vi "set_value.vi"(8 "error in (no error)":errorcluster, 9 "value":variant, 10 "key":string, 11 "Map.lvclass in":refnum<class "Map.lvclass">) -> (0 "error out":errorcluster, 3 "Map.lvclass out":refnum<class "Map.lvclass">)   [LabVIEW 2010, in "Map.lvclass"]
doc: "This method assigns a value to a given key. You can access only direct entry, but not entries further down the hierarchy in the case of a nested map."
uses:
  Map.lvclass
  element_cluster.ctl
  Map.lvclass/Map.ctl
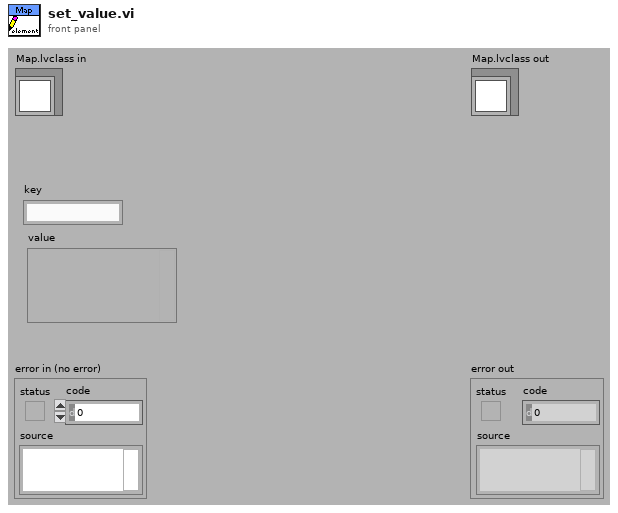
[diagram p1: front panel]
types:
  T1 = typedef "Map.lvclass/element_cluster.ctl" = cluster{"key":string, "value":variant}
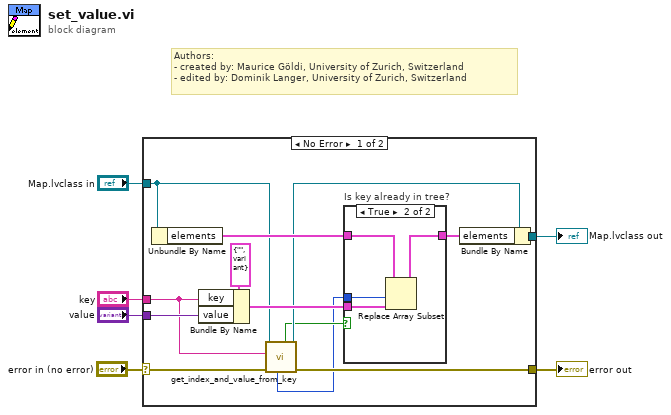
[diagram p0: block diagram]
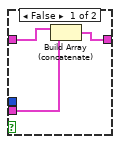
[diagram p2: hidden frame]
diagram:
  # "Authors: \n- created by: Maurice Göldi, University of Zurich, Switzerland\n- edited by: Dominik Langer, University of Zurich, Switzerland"
  n1 = case shown="No Error" "error in (no error)" {
    selector: "error in (no error)" -> [w13 w27]
    tunnel: [w12 w27] -> w5
    tunnel: [w19 w28] -> w3
    tunnel: "Map.lvclass in" -> [w10 w28]
    tunnel: "key" -> [w11 _]
    tunnel: "value" -> [w15 _]
    frame No Error {
      n2 = Unbundle By Name(w10) -> ("elements"=w18:T1[])
      n3 = Bundle By Name(cluster=T1 {"key"="", "value"=variant} ("map_elements"), "key"=w11, "value"=w15) -> (w14:T1)
      n4 = call "get_index_and_value_from_key.vi"("error in (no error)"=w13, "key"=w11, "Map.lvclass in"=w10) -> ("error out"=w12:errorcluster, "Map.lvclass out"=w9:refnum<class "Map.lvclass">, "key exists?"=w8:bool, "index"=w7:i32)  [unwired: 5 out]
      n5 = case "Is key already in tree?" shown="True" w8 {
        tunnel: w18 -> [w22 w26]
        tunnel: [w21 w25] -> w17
        tunnel: w14 -> [w20 w24]
        tunnel: w7 -> [_ w23]
        frame False {
          n6 = Build Array (concatenate)(w22, w20) -> (w21:T1[])
        }
        frame True {
          n7 = Replace Array Subset(array=w26, new element=w24, index=w23) -> (w25:T1[])
        }
      }
      n8 = Bundle By Name(cluster=w9, "elements"=w17) -> (w19:refnum<class "Map.lvclass">)
    }
    frame Error {
    }
  }
  "error out" <- w5
  "Map.lvclass out" <- w3
